vi "Actor Core.vi"(8 "error in":errorcluster, 11 "CRIO MSS Test Actor in":refnum<class "MSS Target Actor.lvclass">) -> (0 "error out":errorcluster, 3 "Actor out":refnum<class "Actor.lvclass">)   [LabVIEW 2023, in "MSS Target Actor.lvlib" / "MSS Target Actor.lvclass"]
doc: "(<B>Filename</B>: Actor Framework.lvlib:Actor.lvclass:Actor Core.vi)\n\nReceives messages to the actor, reacts to them, and initiates any error handling that may shut the actor down.\n\nDescendant classes may override this VI to append parallel tasks for the actor to complete while it handles messages. Overrides use the Call Parent Class Method node."
uses:
  MSS Target Actor.lvclass
  MSS Target Actor.lvclass/MSS Target Actor.ctl
  <vilib>/ni/Actors/Network Endpoint Actors/Notifying Nested Endpoint/Notifying Nested Endpoint.lvclass
  <vilib>/ni/Actors/Network Endpoint Actors/Network Endpoint/Network Endpoint/Network Endpoint.lvclass
  <vilib>/ActorFramework/Actor/Actor.lvclass
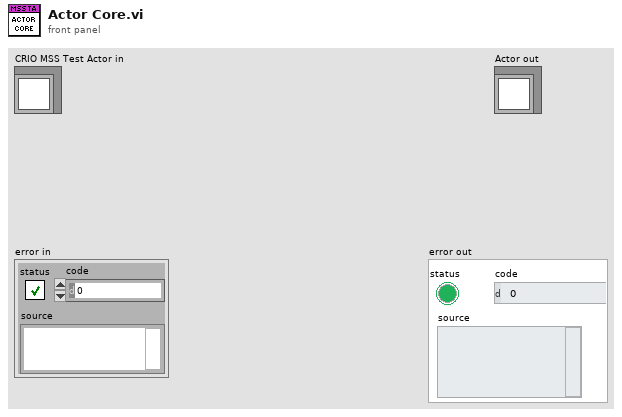
[diagram p1: front panel]
types:
  T1 = map{string, refnum<class "Message Enqueuer.lvclass">}
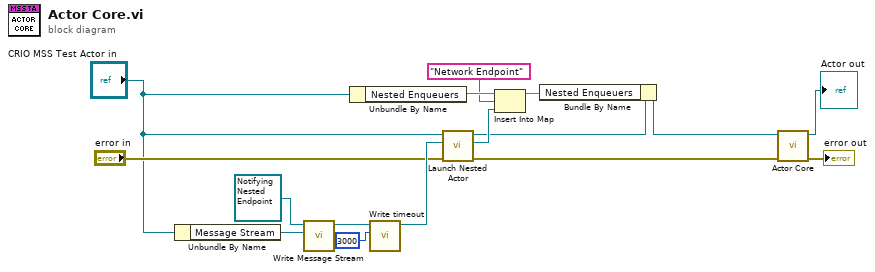
[diagram p0: block diagram]
diagram:
  n1 = Unbundle By Name("CRIO MSS Test Actor in") -> ("Message Stream"=w12:refnum<class "Message Stream.lvclass">)
  n2 = call <vilib>:"Write Message Stream.vi"("Message Stream"=w12, "Network Endpoint in"=refnum<class "Notifying Nested Endpoint.lvclass"> refnum ("Notifying Nested Endpoint.lvclass")) -> ("Network Endpoint out"=w13:refnum<class "Notifying Nested Endpoint.lvclass">)  [unwired: 9 in]
  n3 = Unbundle By Name("CRIO MSS Test Actor in") -> ("Nested Enqueuers"=w9:T1)
  n4 = call <vilib>:"Write timeout.vi"("timeout"=3000, "Network Endpoint in"=w13) -> ("Network Endpoint out"=w10:refnum<class "Notifying Nested Endpoint.lvclass">)  [unwired: 9 in]
  n5 = call <vilib>:"Launch Nested Actor.vi"("error in (no error)"="error in", "Nested Actor"=w10, "Caller Actor in"="CRIO MSS Test Actor in") -> ("error out"=w1:errorcluster, "Nested Actor's Enqueuer"=w7:refnum<class "Message Enqueuer.lvclass">, "Caller Actor out"=w6:refnum<class "MSS Target Actor.lvclass">)  [unwired: 6 in]
  n6 = Insert Into Map(map in=w9, key="Network Endpoint", value=w7) -> (map out=w4:T1)  [unwired: 2 out]
  n7 = Bundle By Name(cluster=w6, "Nested Enqueuers"=w4) -> (w5:refnum<class "MSS Target Actor.lvclass">)
  n8 = call-parent "Actor Core.vi"("error in"=w1, "Actor in"=w5) -> ("error out"=→"error out":errorcluster, "Actor out"=→"Actor out":refnum<class "Actor.lvclass">)  [unwired: 8 in]
